vi "ZoomIn.vi"(0 "reference in":refnum<class "LcPictureBox.lvclass">, 1 "NewScaleValue":dbl, 2 "MousePosition(scaled)":cluster{"X":sgl, "Y":sgl}, 5 "Error In":errorcluster, 6 "ZoomAtMouse":bool=TRUE, 7 "OnlyCaluclateNewValues":bool) -> (14 "reference out":refnum<class "LcPictureBox.lvclass">, 15 "ScaleFactorUsed":dbl=1.0, 16 "Origin":cluster{"x":sgl, "y":sgl}, 19 "Error Out":errorcluster)   [LabVIEW 2020, in "LcPictureBox.lvclass"]
uses:
  LcPictureBox.lvclass
panel:
  out "ScaledMousePos changed after new scale applied":cluster{"Numeric":sgl, "Numeric":sgl}
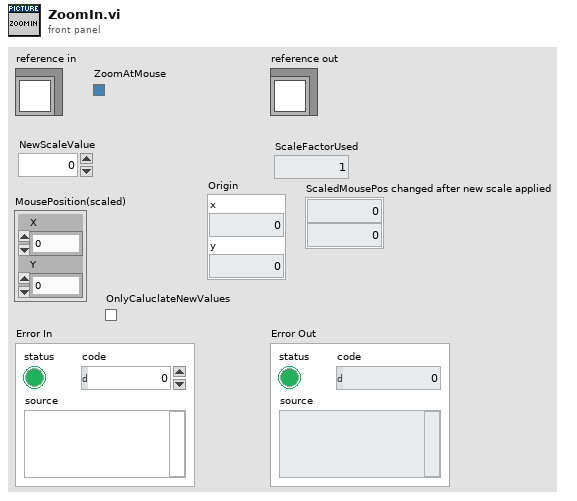
[diagram p1: front panel]
types:
  T1 = typedef "LcPictureBox.lvclass/ObjectAttributes.ctl" = cluster{"PictureBox":refnum<k24>, "ImageSize":cluster{"Width":i32, "Height":i32}, "PenMemory":map{cluster{"Alpha(100%)":dbl, "Color(Black)":u32, "Pen(Width=1, Solid)":T2}, refnum<k24>}, "GraphicsRef":refnum<k24>, "BrushMemory":map{cluster{"Alpha(100%)":dbl, "Color(Black)":u32}, refnum<k24>}, "Images":refnum<k24>[], "ImageIndex":i32, "BgColor(None)":u32, "LoadedImages":map{string, cluster{"ImageOut":refnum<k24>, "ImageSize":cluster{"Width":i32, "Height":i32}}}, "ColorsMemory":map{cluster{"Alpha(100%)":dbl, "Color(Black)":u32}, refnum<k24>}, "CacheSize":i32, "PictureBoxActiveXReference":refnum<vi>, "Scale":dbl, "Offset":cluster{"x":sgl, "y":sgl}, "zoom_center":cluster{"X":i32, "Y":i32}, "ImagesCreated":refnum<k24>[], "CustomCursorImages":map{u16, refnum<k24>}}
  T2 = typedef "LcPictureBox.lvclass/Pen.ctl" = cluster{"Width":u16, "Style":enum32{"Solid", "Dash", "Dot", "DashDot", "DashDotDot"}}
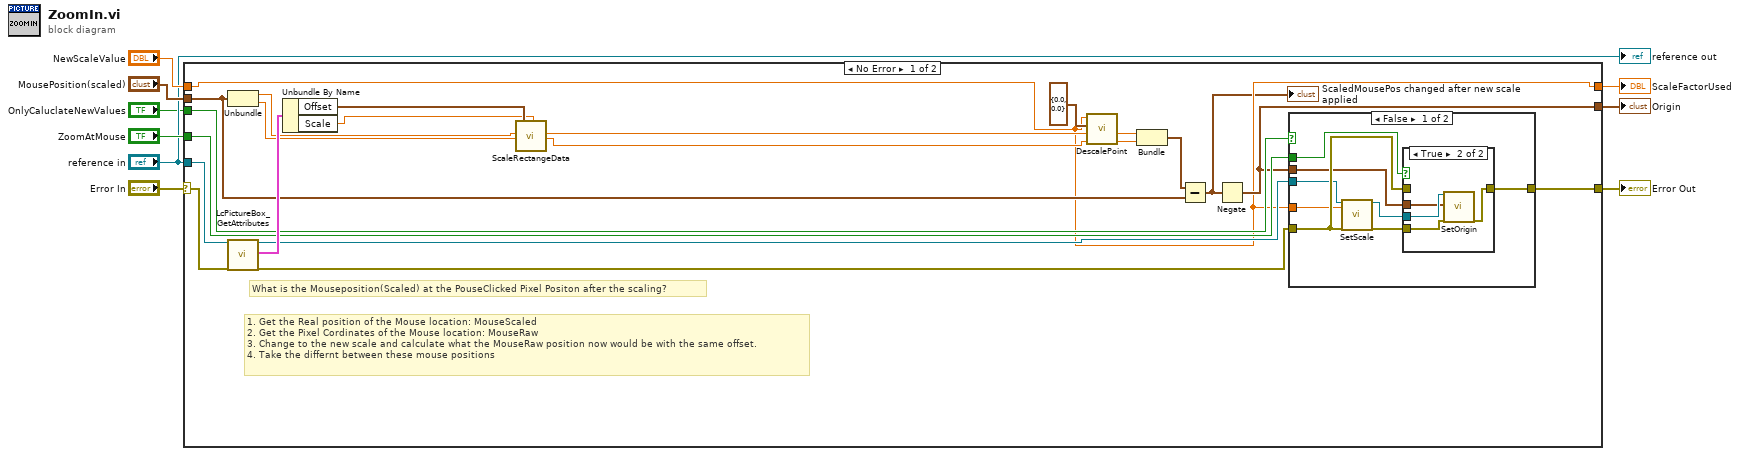
[diagram p0: block diagram]
diagram:
  n1 = case shown="No Error" "Error In" {
    selector: "Error In" -> [w31 w46]
    tunnel: [w27 w46] -> w8
    tunnel: "reference in" -> [w30 _]
    tunnel: "NewScaleValue" -> [w11 _]
    tunnel: "MousePosition(scaled)" -> [w17 _]
    tunnel: "ZoomAtMouse" -> [w26 _]
    tunnel: [w11 _] -> w4
    tunnel: [w22 _] -> w2
    tunnel: "OnlyCaluclateNewValues" -> [w24 _]
    frame No Error {
      # "What is the Mouseposition(Scaled) at the PouseClicked Pixel Positon after the scaling?"
      # "1. Get the Real position of the Mouse location: MouseScaled\n2. Get the Pixel Cordinates of the Mouse location: MouseRaw\n3. Change to the new scale and calculate what the MouseRaw position now would be with the same offset.\n4. Take the differnt between these mouse positions"
      n2 = Unbundle(w17) -> ("X"=w23:sgl, "Y"=w15:sgl)
      n3 = call "LcPictureBox_GetAttributes.vi"("reference in"=w30, "error in (no error)"=w31) -> ("reference out"=w25:refnum<class "LcPictureBox.lvclass">, "Data"=w29:T1, "error out"=w28:errorcluster)  [unwired: 14 in, 1 out]
      n4 = Unbundle By Name(w29) -> ("Offset"=w14:cluster{"x":sgl, "y":sgl}, "Scale"=w13:dbl)
      n5 = call "ScaleRectangeData.vi"("X-In"=w23, "Y-In"=w15, "Offset(raw)"=w14, "Scale"=w13) -> ("X-Out"=w21:sgl, "Y-Out"=w20:sgl)  [unwired: 12 in, 2 out]
      n6 = call "DescalePoint.vi"("Y"=w20, "X"=w21, "Offset"=cluster{"x":dbl, "y":dbl} {"x"=0.0, "y"=0.0}, "Scale"=w11) -> ("Y-Out"=w18:dbl, "X-Out"=w19:dbl)  [unwired: 6 in]
      n7 = Bundle("X-Out"=w19, "Y-Out"=w18) -> (w16:cluster{"X-Out":dbl, "Y-Out":dbl})  [unwired: 1 in]
      n8 = Subtract(x=w16, y=w17) -> (x-y=w10:cluster{dbl, dbl})
      "ScaledMousePos changed after new scale applied" <- w10
      n9 = Negate(x=w10) -> (-x=w22:cluster{dbl, dbl})
      n10 = case shown="False" w24 {
        tunnel: w28 -> [w39 w45]
        tunnel: [w38 w45] -> w27
        tunnel: w11 -> [w37 _]
        tunnel: w26 -> [w36 _]
        tunnel: w25 -> [w35 _]
        tunnel: w22 -> [w32 _]
        frame False {
          n11 = call-dynamic "SetScale.vi"("reference in"=w35, "ScaleFactor"=w37, "Error In"=w39) -> ("reference out"=w34:refnum<class "LcPictureBox.lvclass">, "Error Out"=w33:errorcluster)  [unwired: 15 in]
          n12 = case shown="True" w36 {
            tunnel: w39 -> [w40 _]
            tunnel: [w40 w44] -> w38
            tunnel: w34 -> [_ w43]
            tunnel: w33 -> [_ w42]
            tunnel: w32 -> [_ w41]
            frame False {
            }
            frame True {
              n13 = call-dynamic "SetOrigin.vi"("reference in"=w43, "Origin"=w41, "Error In"=w42) -> ("Error Out"=w44:errorcluster)  [unwired: 15 in, 1 out]
            }
          }
        }
        frame True {
        }
      }
    }
    frame Error {
    }
  }
  "Error Out" <- w8
  "ScaleFactorUsed" <- w4
  "Origin" <- w2
  "reference out" <- "reference in"
